vi "Introspection Core.vi"(8 "error in (no error)":errorcluster, 11 "IVI_Counter in":refnum<class "IVI_Counter.lvclass">) -> (0 "error out":errorcluster, 2 "CS++Messages":refnum<class "Message.lvclass">[](array[class]), 3 "IVI_Counter out":refnum<class "IVI_Counter.lvclass">)   [LabVIEW 2014, in "IVI_Counter.lvlib" / "IVI_Counter.lvclass"]
doc: "This vi delivers a list with all messages this actor reacts to. \n\nNote that all inherited classes have to overwrite it."
uses:
  IVI_Counter.lvclass
  <vilib>/ActorFramework/Message/Message.lvclass
  CSPP_Core/Actors/CS++DeviceActor/CS++DeviceActor.lvclass
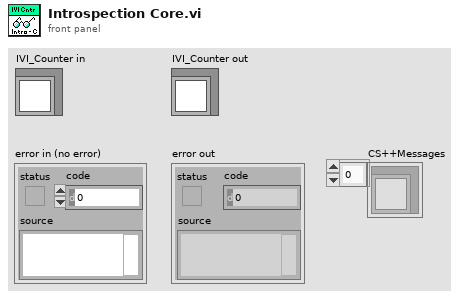
[diagram p1: front panel]
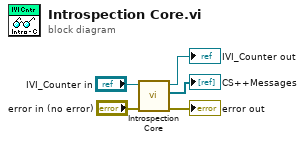
[diagram p0: block diagram]
diagram:
  n1 = call-parent "Introspection Core.vi"("error in (no error)"="error in (no error)", "CS++DeviceActor in"="IVI_Counter in") -> ("error out"=→"error out":errorcluster, "CS++Messages"=→"CS++Messages":refnum<class "Message.lvclass">[], "CS++DeviceActor out"=→"IVI_Counter out":refnum<class "IVI_Counter.lvclass">)  [unwired: 7 in]
